vi "GDSLvIcon_FindIconSplitter.vi"(9 "Icon(Top Frame Rows removed)":u8[][](array[numeric]), 10 "SolidTopRow'sMost Common Color)":u8[](array[numeric]), 11 "TopRow(Frame)":u8[](array[numeric])) -> (2 "Splitter probably found":bool, 3 "Splitter Index found (-(FrameThickness), since the Icon in is missing the Frame)":i32)   [LabVIEW 2020]
uses:
  <vilib>/Analysis/NI_AALBase.lvlib
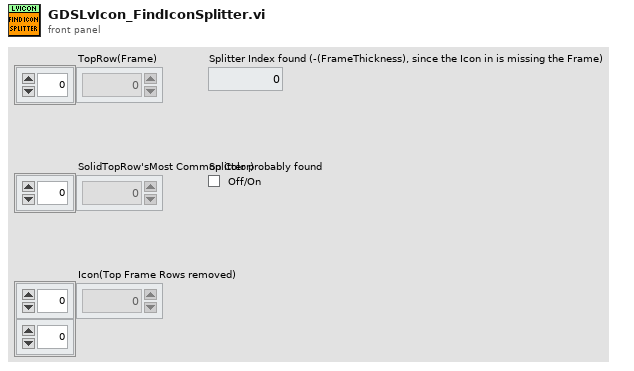
[diagram p1: front panel]
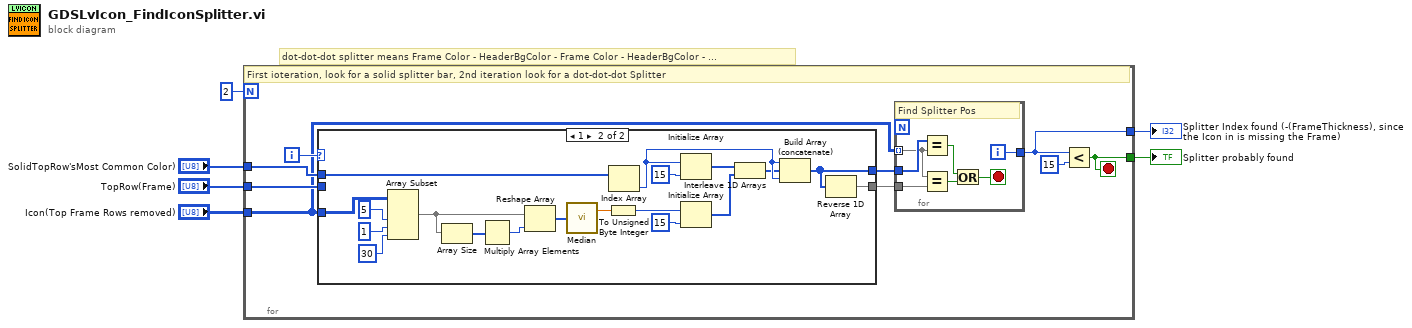
[diagram p0: block diagram]
diagram:
  # "dot-dot-dot splitter means Frame Color - HeaderBgColor - Frame Color - HeaderBgColor - ..."
  n1 = for {
    N: 2 -> [_]
    tunnel: [w15] -> w6
    tunnel: [w13] -> w5
    tunnel: "Icon(Top Frame Rows removed)" -> [w7]
    tunnel: "TopRow(Frame)" -> [w10]
    tunnel: "SolidTopRow'sMost Common Color)" -> [w11]
    i -> [w12]
    stop <- w13 stop-if-true
    # "First ioteration, look for a solid splitter bar, 2nd iteration look for a dot-dot-dot Splitter"
    n2 = case shown="1" w12 {
      tunnel: w11 -> [w16 w36]
      tunnel: w10 -> [w17 _]
      tunnel: [w17 w18] -> w9
      tunnel: [w16 w19] -> w8
      tunnel: w7 -> [_ w35]
      frame 0, Default {
      }
      frame 1 {
        n3 = Array Subset(array=w35, length (row)=5 ("length"), index (col)=1 ("index"), length (col)=30 ("length")) -> (w31:u8[][])  [unwired: 1 in]
        n4 = Array Size(array=w31) -> (size(s)=w30:i32[])
        n5 = Multiply Array Elements(1:w30) -> (0:w29:i32)
        n6 = Reshape Array(w31, w29) -> (w28:u8[])
        n7 = call <vilib>:"Median.vi"("X"=w28) -> ("median"=w25:dbl)  [unwired: 1 out]
        n8 = To Unsigned Byte Integer(number=w25) -> (unsigned 8bit integer=w24:u8)
        n9 = Index Array(array=w36) -> (element=w21:u8)  [unwired: 1 in]
        n10 = Initialize Array(w21, 15 ("dimension size")) -> (w23:u8[])
        n11 = Initialize Array(w24, 15 ("dimension size")) -> (w22:u8[])
        n12 = Interleave 1D Arrays(w23, w22) -> (w20:u8[])
        n13 = Build Array (concatenate)(w21, w20, w21) -> (w19:u8[])
        n14 = Reverse 1D Array(array=w19) -> (reversed array=w18:u8[])
      }
    }
    n15 = for {
      tunnel: w7 -> [w41] mode=indexing
      tunnel: w8 -> [w43]
      tunnel: [w42] -> w15
      tunnel: w9 -> [w40]
      i -> [w42]
      stop <- w37 stop-if-true
      # "Find Splitter Pos"
      n16 = Equal?(x=w43, y=w41) -> (x = y?=w39:bool)
      n17 = Equal?(x=w41, y=w40) -> (x = y?=w38:bool)
      n18 = Or(x=w39, y=w38) -> (x .or. y?=w37:bool)
    }
    n19 = Less?(x=w15, y=15) -> (x < y?=w13:bool)
  }
  "Splitter Index found (-(FrameThickness), since the Icon in is missing the Frame)" <- w6
  "Splitter probably found" <- w5
